vi "WritingDataBaseDataToFiles.vi"() -> ()   [LabVIEW 2019]
uses:
  <vilib>/addons/database/Recordset.llb/Rec Save Format.ctl
  <vilib>/addons/database/Connection.llb/DB Tools Open Connec (String).vi
  <vilib>/addons/database/Connection.llb/Conn Execute.vi
  <vilib>/addons/database/Recordset.llb/Rec Save Recordset To File (R).vi
  <vilib>/addons/database/Recordset.llb/Rec Destroy - Connection.vi
  <vilib>/addons/database/NI_Database_API.lvlib
panel:
  in  "Provide Your ODBC server Name here":string
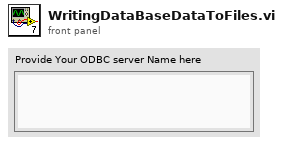
[diagram p1: front panel]
types:
  T1 = typedef "NI_Database_API.lvlib/Rec Save Format.ctl" = enum16{"ADTG", "XML"}
  T2 = typedef "NI_Database_API.lvlib/Conn ObjectReference.ctl" = refnum<k1>
  T3 = typedef "NI_Database_API.lvlib/Rec ObjectReference.ctl" = refnum<k1>
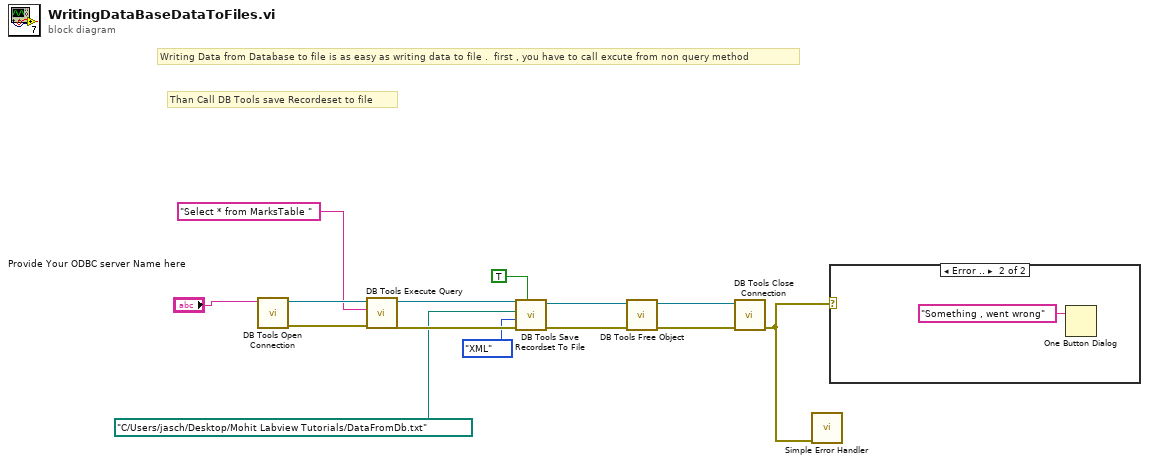
[diagram p0: block diagram]
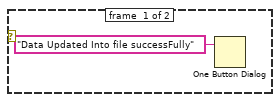
[diagram p2: hidden frame]
diagram:
  # "Than Call DB Tools save Recordeset to file"
  # "Writing Data from Database to file is as easy as writing data to file .  first , you have to call excute from non query method"
  n1 = call-poly <vilib>:"DB Tools Open Connection.vi"("connection information"="Provide Your ODBC server Name here") -> ("error out"=w12:errorcluster, "connection reference"=w13:T2)  [unwired: 7 in]
  n2 = call-poly <vilib>:"DB Tools Execute Query.vi"("error in (no error)"=w12, "SQL query"="Select * from MarksTable ", "connection reference"=w13) -> ("error out"=w10:errorcluster, "recordset reference"=w9:T3)  [unwired: 5 in]
  n3 = call-poly <vilib>:"DB Tools Save Recordset To File.vi"("overwrite? (F)"=TRUE, "error in (no error)"=w10, "save format (XML)"=Rec_Save_Format."XML", "file name"=path "C:/Users/jasch/Desktop/Mohit Labview Tutorials/DataFromDb.txt", "recordset reference"=w9) -> ("error out"=w6:errorcluster, "recordset reference out"=w7:T3)  [unwired: 3 in]
  n4 = call-poly <vilib>:"DB Tools Free Object.vi"("error in (no error)"=w6, "recordset reference"=w7) -> ("error out"=w4:errorcluster, "connection reference"=w5:T2)  [unwired: 8 in]
  n5 = call <vilib>:"DB Tools Close Connection.vi"("error in (no error)"=w4, "connection reference"=w5) -> ("error out"=w3:errorcluster)  [unwired: 5 in]
  n6 = call <vilib>:"Simple Error Handler.vi"("error in (no error)"=w3) -> ()  [unwired: 4 in, 5 out]
  n7 = case shown="Error .." w3 {
    frame #0 {
      n8 = One Button Dialog(message="Data Updated Into file successFully") -> ()  [unwired: 1 in, 1 out]
    }
    frame #1 {
      n9 = One Button Dialog(message="Something , went wrong") -> ()  [unwired: 1 in, 1 out]
    }
  }
